vi "Main Dialog.vi"(8 "error in (no error)":errorcluster, 11 "New Class Dialog In":refnum<class "New Class Dialog.lvclass">) -> (0 "error out":errorcluster, 3 "New Class Dialog Out":refnum<class "New Class Dialog.lvclass">)   [LabVIEW 2020, in "New Class Dialog.lvclass"]
uses:
  New Class Dialog.lvclass
  Helpers/Tag Tree Helper/Tag Tree Helper.lvclass
  Helpers/Tag Tree Helper/Tag Tree Helper.lvclass/Tag Tree Helper.ctl
  New Class Dialog.lvclass/New Class Dialog.ctl
  Class Generation/Process Generator/Process Generator.lvclass/Process Generator.ctl
  Class Generation/Process Generator/Process Generator.lvclass
panel:
  in  "Parent Class":string(tree)
  in  "Process Name":string
  in  "Save to Folder":path
  in  "Commit":bool
  in  "Cancel":bool
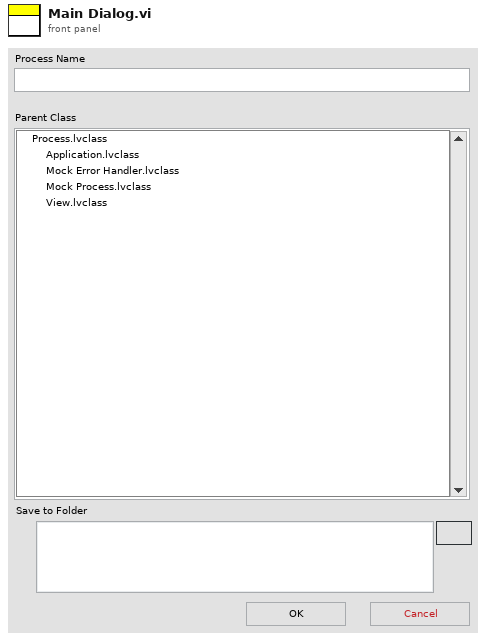
[diagram p1: front panel]
types:
  T1 = enum8{"Enabled", "Disabled", "Disabled and Grayed Out"}
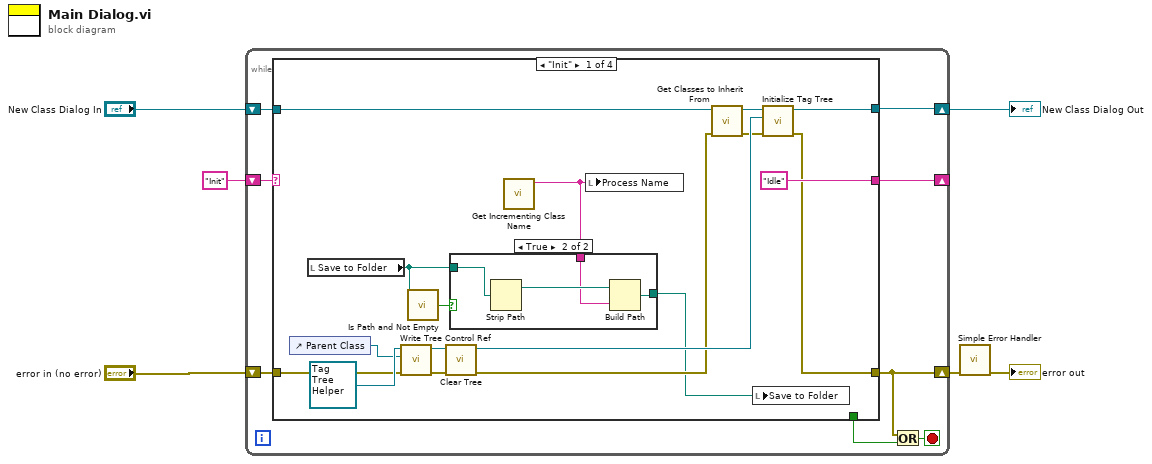
[diagram p0: block diagram]
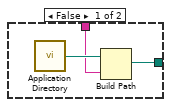
[diagram p2: hidden frame]
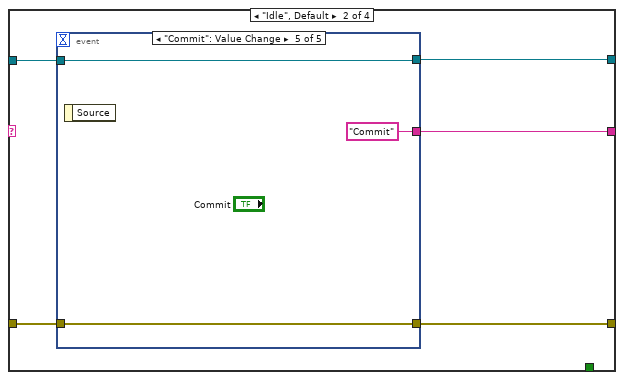
[diagram p3: hidden frame]
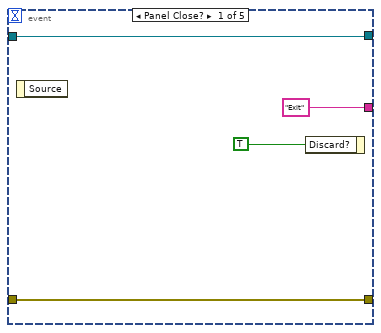
[diagram p4: hidden frame]
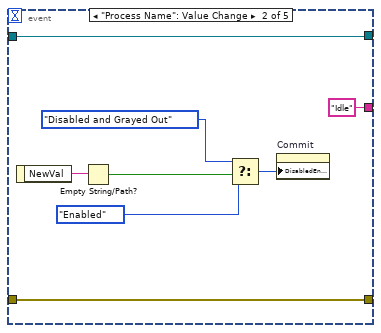
[diagram p5: hidden frame]
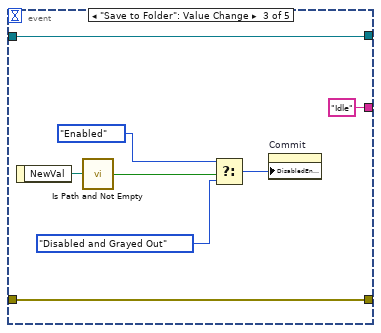
[diagram p6: hidden frame]
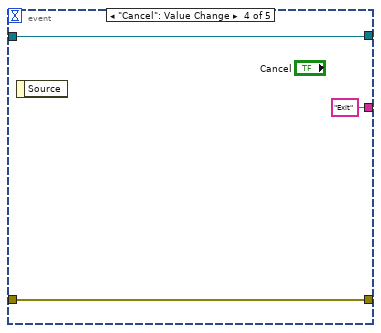
[diagram p7: hidden frame]
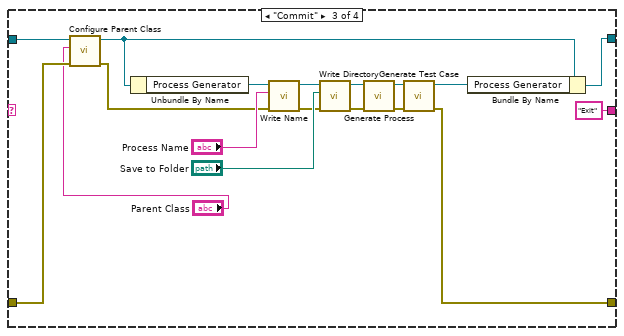
[diagram p8: hidden frame]
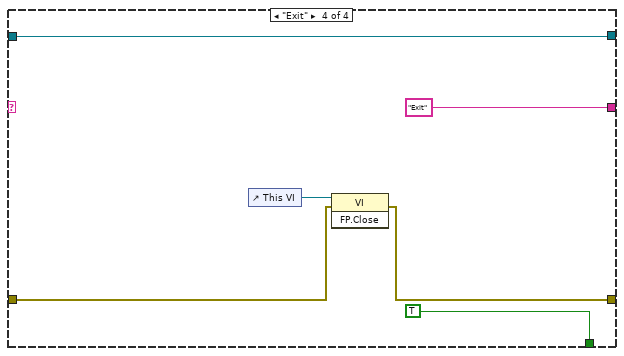
[diagram p9: hidden frame]
diagram:
  n1 = while {
    shift-right: [w11] -> w4
    shift-left: "New Class Dialog In" -> [w12]
    shift-right: [w7] -> w3
    shift-left: "error in (no error)" -> [w13]
    shift-right: [w10] -> _
    shift-left: "Init" -> [w14]
    stop <- w8 stop-if-true
    n2 = case shown="\"Init\"" w14 {
      tunnel: [w24 w43 w74 w89] -> w7
      tunnel: w13 -> [w21 w42 w76 w88]
      tunnel: w12 -> [w30 w41 w72 w93]
      tunnel: [w26 w40 w75 w93] -> w11
      tunnel: ["Idle" w39 "Exit" "Exit"] -> w10
      tunnel: [_ _ _ TRUE] -> w9
      frame "Init" {
        n3 = control-ref of="Parent Class"() -> (w28:refnum<vi>)
        n4 = local read "Save to Folder"() -> (w18:path)
        n5 = call "Write Tree Control Ref.vi"("error in (no error)"=w21, "Tag Tree Reference"=w28, "Tag Tree Helper In"=refnum<class "Tag Tree Helper.lvclass"> refnum ("Support Utilities.lvlib:Tag Tree.lvclass")) -> ("error out"=w25:errorcluster, "Tag Tree Helper Out"=w22:refnum<class "Tag Tree Helper.lvclass">)  [unwired: 7 in]
        n6 = call <vilib>:"Is Path and Not Empty.vi"("path"=w18) -> ("Is Path and Not Empty?"=w16:bool)  [unwired: 4 in]
        n7 = call "Clear Tree.vi"("error in (no error)"=w25, "Tag Tree Helper In"=w22) -> ("error out"=w20:errorcluster, "Tag Tree Helper Out"=w23:refnum<class "Tag Tree Helper.lvclass">)  [unwired: 8 in]
        n8 = call "Get Incrementing Class Name.vi"() -> ("String"=w17:string)  [unwired: 11 in]
        n9 = case shown="True" w16 {
          tunnel: w18 -> [_ w38]
          tunnel: w17 -> [w33 w36]
          tunnel: [w32 w35] -> w15
          frame False {
            n10 = call <vilib>:"Application Directory.vi"() -> ("Application Directory"=w34:path)
            n11 = Build Path(base path=w34, name or relative path=w33) -> (appended path=w32:path)
          }
          frame True {
            n12 = Strip Path(path=w38) -> (stripped path=w37:path)  [unwired: 1 out]
            n13 = Build Path(base path=w37, name or relative path=w36) -> (appended path=w35:path)
          }
        }
        n14 = local write "Process Name"(w17) -> ()
        n15 = call "Get Classes to Inherit From.vi"("error in (no error)"=w20, "New Class Dialog In"=w30) -> ("error out"=w19:errorcluster, "New Class Dialog Out"=w27:refnum<class "New Class Dialog.lvclass">)  [unwired: 8 in]
        n16 = local write "Save to Folder"(w15) -> ()
        n17 = call "Initialize Tag Tree.vi"("error in (no error)"=w19, "Tag Tree Helper"=w23, "New Class Dialog In"=w27) -> ("error out"=w24:errorcluster, "New Class Dialog Out"=w26:refnum<class "New Class Dialog.lvclass">)  [unwired: 7 in]
      }
      frame "Idle", Default {
        n18 = event shown="[4] \"Commit\": Value Change" {
          selector: _ -> [_ _ _ _ _]
          dyn-events: _ -> [_ _ _ _ _]
          timeout: _ -> [_ _ _ _ _]
          tunnel: [w47 w55 w63 w65 w69] -> w43
          tunnel: w42 -> [w47 w55 w63 w65 w69]
          tunnel: w41 -> [w46 w54 w62 w66 w68]
          tunnel: [w46 w54 w62 w66 w68] -> w40
          tunnel: ["Exit" "Idle" "Idle" "Exit" "Commit"] -> w39
          event Panel Close? {
            n19 = event-data() -> ()  [unwired: 1 in, 1 out]
            n20 = event-data("Discard?"=TRUE) -> ()  [unwired: 1 in, 1 out]
          }
          event "Process Name": Value Change {
            n21 = event-data() -> ("NewVal"=w53:string)  [unwired: 1 in]
            n22 = Empty String/Path?(string/path=w53) -> (empty?=w52:bool)
            n23 = Select(t=T1."Disabled and Grayed Out" ("Disabled"), s=w52, f=T1."Enabled") -> (s? t:f=w49:T1)
            n24 = property on="Commit" class="Bool"("DisabledEnum"=w49) -> ()  [unwired: 2 in, 2 out]
          }
          event "Save to Folder": Value Change {
            n25 = event-data() -> ("NewVal"=w61:path)  [unwired: 1 in]
            n26 = call <vilib>:"Is Path and Not Empty.vi"("path"=w61) -> ("Is Path and Not Empty?"=w60:bool)  [unwired: 4 in]
            n27 = Select(t=T1."Enabled" ("f"), s=w60, f=T1."Disabled and Grayed Out" ("Disabled")) -> (s? t:f=w57:T1)
            n28 = property on="Commit" class="Bool"("DisabledEnum"=w57) -> ()  [unwired: 2 in, 2 out]
          }
          event "Cancel": Value Change {
            n29 = event-data() -> ()  [unwired: 1 in, 1 out]
          }
          event "Commit": Value Change {
            n30 = event-data() -> ()  [unwired: 1 in, 1 out]
          }
        }
      }
      frame "Commit" {
        n31 = call "Configure Parent Class.vi"("error in (no error)"=w76, "Parent Class"="Parent Class", "New Class Dialog In"=w72) -> ("error out"=w73:errorcluster, "New Class Dialog Out"=w71:refnum<class "New Class Dialog.lvclass">)  [unwired: 7 in]
        n32 = Unbundle By Name(w71) -> ("Process Generator"=w84:refnum<class "Process Generator.lvclass">)
        n33 = call "Write Name.vi"("error in (no error)"=w73, "Name"="Process Name", "Process Generator In"=w84) -> ("error out"=w82:errorcluster, "Process Generator Out"=w83:refnum<class "Process Generator.lvclass">)  [unwired: 7 in]
        n34 = call "Write Directory.vi"("error in (no error)"=w82, "Directory"="Save to Folder", "Process Generator in"=w83) -> ("error out"=w80:errorcluster, "Process Generator out"=w81:refnum<class "Process Generator.lvclass">)  [unwired: 7 in]
        n35 = call "Generate Process.vi"("error in (no error)"=w80, "Process Generator In"=w81) -> ("error out"=w78:errorcluster, "Process Generator Out"=w79:refnum<class "Process Generator.lvclass">)  [unwired: 8 in]
        n36 = call "Generate Test Case.vi"("error in (no error)"=w78, "Process Generator In"=w79) -> ("error out"=w74:errorcluster, "Process Generator Out"=w77:refnum<class "Process Generator.lvclass">)  [unwired: 8 in]
        n37 = Bundle By Name(cluster=w71, "Process Generator"=w77) -> (w75:refnum<class "New Class Dialog.lvclass">)
      }
      frame "Exit" {
        n38 = control-ref of="This VI"() -> (w90:refnum<vi>)
        n39 = invoke class="VI" method="FP.Close"(reference=w90, error in=w88) -> (error out=w89:errorcluster)  [unwired: 1 in, 2 out]
      }
    }
    n40 = Or(x=w7, y=w9) -> (x .or. y?=w8:bool)
  }
  "New Class Dialog Out" <- w4
  n41 = call <vilib>:"Simple Error Handler.vi"("error in (no error)"=w3) -> ("error out"=→"error out":errorcluster)  [unwired: 4 in, 4 out]
